vi "Encoder Crossover.vi"(4 "Previous Value 2":dbl, 5 "Previous Value":dbl, 6 "Encoder Value 2":dbl, 7 "Encoder Value":dbl) -> (0 "Encoder Output 2":dbl, 1 "Encoder Output":dbl)   [LabVIEW 2015]
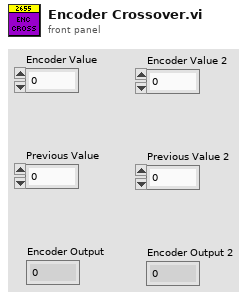
[diagram p1: front panel]
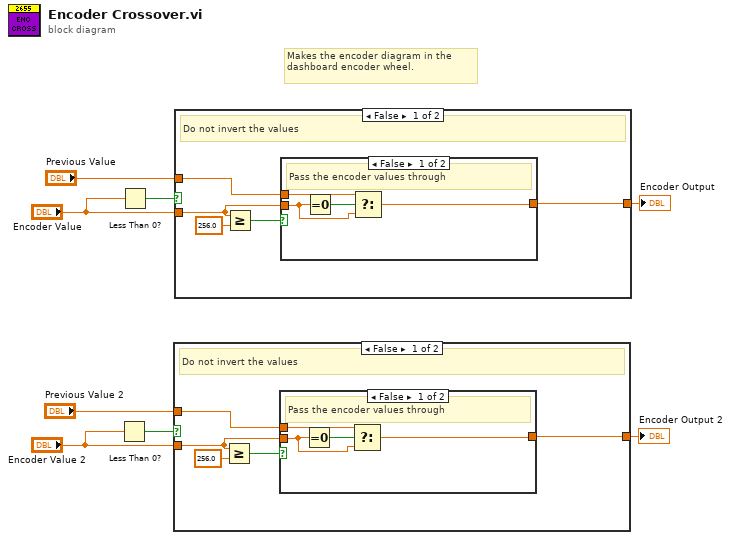
[diagram p0: block diagram]
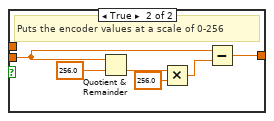
[diagram p2: hidden frame]
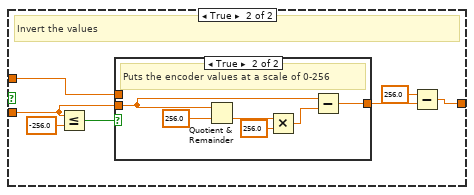
[diagram p3: hidden frame]
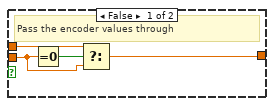
[diagram p4: hidden frame]
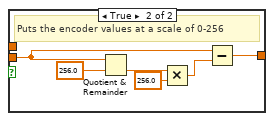
[diagram p5: hidden frame]
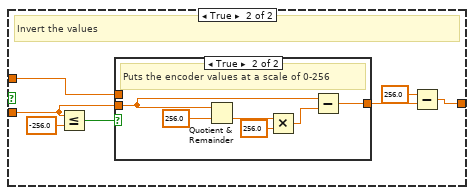
[diagram p6: hidden frame]
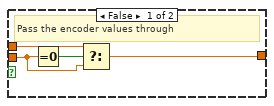
[diagram p7: hidden frame]
diagram:
  # "Makes the encoder diagram in the dashboard encoder wheel."
  n1 = Less Than 0?(x="Encoder Value 2") -> (x < 0?=w2:bool)
  n2 = Less Than 0?(x="Encoder Value") -> (x < 0?=w6:bool)
  n3 = case shown="False" w2 {
    tunnel: "Previous Value 2" -> [w11 w27]
    tunnel: "Encoder Value 2" -> [w10 w28]
    tunnel: [w9 w24] -> w1
    frame False {
      # "Do not invert the values"
      n4 = Greater Or Equal?(x=w10, y=256.0) -> (x >= y?=w13:bool)
      n5 = case shown="False" w13 {
        tunnel: w10 -> [w15 w20]
        tunnel: [w14 w21] -> w9
        tunnel: w11 -> [w16 _]
        frame False {
          # "Pass the encoder values through"
          n6 = Equal To 0?(x=w15) -> (x = 0?=w17:bool)
          n7 = Select(t=w16, s=w17, f=w15) -> (s? t:f=w14:dbl)
        }
        frame True {
          # "Puts the encoder values at a scale of 0-256"
          n8 = Quotient & Remainder(x=w20, y=256.0) -> (floor(x/y)=w18:dbl)  [unwired: 1 out]
          n9 = Multiply(x=w18, y=256.0) -> (x*y=w22:dbl)
          n10 = Subtract(x=w20, y=w22) -> (x-y=w21:dbl)
        }
      }
    }
    frame True {
      # "Invert the values"
      n11 = Less Or Equal?(x=w28, y=-256.0) -> (x <= y?=w30:bool)
      n12 = case shown="True" w30 {
        tunnel: w28 -> [w32 w37]
        tunnel: [w31 w38] -> w26
        tunnel: w27 -> [w33 _]
        frame False {
          # "Pass the encoder values through"
          n13 = Equal To 0?(x=w32) -> (x = 0?=w34:bool)
          n14 = Select(t=w33, s=w34, f=w32) -> (s? t:f=w31:dbl)
        }
        frame True {
          # "Puts the encoder values at a scale of 0-256"
          n15 = Quotient & Remainder(x=w37, y=256.0) -> (floor(x/y)=w35:dbl)  [unwired: 1 out]
          n16 = Multiply(x=w35, y=256.0) -> (x*y=w39:dbl)
          n17 = Subtract(x=w37, y=w39) -> (x-y=w38:dbl)
        }
      }
      n18 = Subtract(x=256.0, y=w26) -> (x-y=w24:dbl)
    }
  }
  "Encoder Output 2" <- w1
  n19 = case shown="False" w6 {
    tunnel: "Previous Value" -> [w43 w59]
    tunnel: "Encoder Value" -> [w42 w60]
    tunnel: [w41 w56] -> w5
    frame False {
      # "Do not invert the values"
      n20 = Greater Or Equal?(x=w42, y=256.0) -> (x >= y?=w45:bool)
      n21 = case shown="False" w45 {
        tunnel: w42 -> [w47 w52]
        tunnel: [w46 w53] -> w41
        tunnel: w43 -> [w48 _]
        frame False {
          # "Pass the encoder values through"
          n22 = Equal To 0?(x=w47) -> (x = 0?=w49:bool)
          n23 = Select(t=w48, s=w49, f=w47) -> (s? t:f=w46:dbl)
        }
        frame True {
          # "Puts the encoder values at a scale of 0-256"
          n24 = Quotient & Remainder(x=w52, y=256.0) -> (floor(x/y)=w50:dbl)  [unwired: 1 out]
          n25 = Multiply(x=w50, y=256.0) -> (x*y=w54:dbl)
          n26 = Subtract(x=w52, y=w54) -> (x-y=w53:dbl)
        }
      }
    }
    frame True {
      # "Invert the values"
      n27 = Less Or Equal?(x=w60, y=-256.0) -> (x <= y?=w62:bool)
      n28 = case shown="True" w62 {
        tunnel: w60 -> [w64 w69]
        tunnel: [w63 w70] -> w58
        tunnel: w59 -> [w65 _]
        frame False {
          # "Pass the encoder values through"
          n29 = Equal To 0?(x=w64) -> (x = 0?=w66:bool)
          n30 = Select(t=w65, s=w66, f=w64) -> (s? t:f=w63:dbl)
        }
        frame True {
          # "Puts the encoder values at a scale of 0-256"
          n31 = Quotient & Remainder(x=w69, y=256.0) -> (floor(x/y)=w67:dbl)  [unwired: 1 out]
          n32 = Multiply(x=w67, y=256.0) -> (x*y=w71:dbl)
          n33 = Subtract(x=w69, y=w71) -> (x-y=w70:dbl)
        }
      }
      n34 = Subtract(x=256.0, y=w58) -> (x-y=w56:dbl)
    }
  }
  "Encoder Output" <- w5
